vi "XY Graph Plot Convolution Dialog.vi"(6 "Reference Decay":cluster{"t Array":dbl[], "I Array":dbl[]}, 8 "Error In":errorcluster, 9 "Valid Reference Decay?":bool, 10 "Plot at Coordinates":i32, 11 "XY Graph":refnum<vi>) -> (0 "Error Out":errorcluster, 1 "Plot Destination out":T4, 2 "Convolution Product Options out":T1 {"Plot 2" items=["M0_H00_000: Plot", "M0_H00_020: Plot"]; "Plot 1" items=["M0_H00_000: Plot", "M0_H00_020: Plot"]}, 3 "XY Graph (dup)":refnum<vi>, 4 "Cancelled":bool)   [LabVIEW 2021, in "XY Graph Add-Ons.lvlib"]
uses:
  Plot Destination.ctl
  XY Graph Convolution Product Options.ctl
  XY Graph Convolution Period Type.ctl
  XY Graph Convolution Step Type.ctl
  XY Graph Add-Ons.lvlib
  Graphs.lvlib
panel:
  in  "Convolution Product Options":T1 {"Step" min=0.0; "Period" min=0.0; "Plot 2" items=["Extrapolated M0 IRF", "M0_H00_000: Liver", "2-Exp Fit of M0_H00_000: Liver", "2-Exp Fit of M0_H00_000: Liver Residuals", "M0_H00_001: Liver", "2-Exp Fit of M0_H00_001: Liver", "2-Exp Fit of M0_H00_001: Liver Residuals", "M0_H00_002: Liver", "2-Exp Fit of M0_H00_002: Liver", "2-Exp Fit of M0_H00_002: Liver Residuals", "M0_H00_003: Liver", "2-Exp Fit of M0_H00_003: Liver", "2-Exp Fit of M0_H00_003: Liver Residuals", "M0_H00_004: Liver", "2-Exp Fit of M0_H00_004: Liver", "2-Exp Fit of M0_H00_004: Liver Residuals", "M0_H00_005: Liver", "2-Exp Fit of M0_H00_005: Liver", "2-Exp Fit of M0_H00_005: Liver Residuals", "M0_H00_006: Liver", "2-Exp Fit of M0_H00_006: Liver", "2-Exp Fit of M0_H00_006: Liver Residuals", "M0_H00_007: Liver", "2-Exp Fit of M0_H00_007: Liver", "2-Exp Fit of M0_H00_007: Liver Residuals", "M0_H00_008: Liver", "2-Exp Fit of M0_H00_008: Liver", "2-Exp Fit of M0_H00_008: Liver Residuals", "M0_H00_009: Liver", "2-Exp Fit of M0_H00_009: Liver", "2-Exp Fit of M0_H00_009: Liver Residuals", "M0_H00_010: Liver", "2-Exp Fit of M0_H00_010: Liver", "2-Exp Fit of M0_H00_010: Liver Residuals", "M0_H00_011: Liver", "2-Exp Fit of M0_H00_011: Liver", "2-Exp Fit of M0_H00_011: Liver Residuals", "M0_H00_012: Liver", "2-Exp Fit of M0_H00_012: Liver", "2-Exp Fit of M0_H00_012: Liver Residuals", "M0_H00_013: Liver", "2-Exp Fit of M0_H00_013: Liver", "2-Exp Fit of M0_H00_013: Liver Residuals", "M0_H00_014: Liver", "2-Exp Fit of M0_H00_014: Liver", "2-Exp Fit of M0_H00_014: Liver Residuals", "M0_H00_015: Liver", "2-Exp Fit of M0_H00_015: Liver", "2-Exp Fit of M0_H00_015: Liver Residuals", "M0_H00_016: Liver", "2-Exp Fit of M0_H00_016: Liver", "2-Exp Fit of M0_H00_016: Liver Residuals", "M0_H00_017: Liver", "2-Exp Fit of M0_H00_017: Liver", "2-Exp Fit of M0_H00_017: Liver Residuals", "M0_H00_018: Liver", "2-Exp Fit of M0_H00_018: Liver", "2-Exp Fit of M0_H00_018: Liver Residuals", "M0_H00_019: Liver", "2-Exp Fit of M0_H00_019: Liver", "2-Exp Fit of M0_H00_019: Liver Residuals", "M0_H00_020: Liver", "2-Exp Fit of M0_H00_020: Liver", "2-Exp Fit of M0_H00_020: Liver Residuals", "M0_H00_021: Liver", "2-Exp Fit of M0_H00_021: Liver", "2-Exp Fit of M0_H00_021: Liver Residuals", "M0_H00_022: Liver", "2-Exp Fit of M0_H00_022: Liver", "2-Exp Fit of M0_H00_022: Liver Residuals", "M0_H00_023: Liver", "2-Exp Fit of M0_H00_023: Liver", "2-Exp Fit of M0_H00_023: Liver Residuals", "M0_H00_024: Liver", "2-Exp Fit of M0_H00_024: Liver", "2-Exp Fit of M0_H00_024: Liver Residuals", "M0_H00_025: Liver", "2-Exp Fit of M0_H00_025: Liver", "2-Exp Fit of M0_H00_025: Liver Residuals", "M0_H00_026: Liver", "2-Exp Fit of M0_H00_026: Liver", "2-Exp Fit of M0_H00_026: Liver Residuals", "M0_H00_027: Liver", "2-Exp Fit of M0_H00_027: Liver", "2-Exp Fit of M0_H00_027: Liver Residuals", "M0_H00_028: Liver", "2-Exp Fit of M0_H00_028: Liver", "2-Exp Fit of M0_H00_028: Liver Residuals", "M0_H00_029: Liver", "2-Exp Fit of M0_H00_029: Liver", "2-Exp Fit of M0_H00_029: Liver Residuals", "M0_H00_030: Liver", "2-Exp Fit of M0_H00_030: Liver", "2-Exp Fit of M0_H00_030: Liver Residuals", "M0_H00_031: Liver", "2-Exp Fit of M0_H00_031: Liver", "2-Exp Fit of M0_H00_031: Liver Residuals", "M0_H00_032: Liver", "2-Exp Fit of M0_H00_032: Liver", "2-Exp Fit of M0_H00_032: Liver Residuals", "M0_H00_033: Liver", "2-Exp Fit of M0_H00_033: Liver", "2-Exp Fit of M0_H00_033: Liver Residuals", "M0_H00_034: Liver", "2-Exp Fit of M0_H00_034: Liver", "2-Exp Fit of M0_H00_034: Liver Residuals", "M0_H00_035: Liver", "2-Exp Fit of M0_H00_035: Liver", "2-Exp Fit of M0_H00_035: Liver Residuals", "M0_H00_036: Liver", "2-Exp Fit of M0_H00_036: Liver", "2-Exp Fit of M0_H00_036: Liver Residuals", "M0_H00_037: Liver", "2-Exp Fit of M0_H00_037: Liver", "2-Exp Fit of M0_H00_037: Liver Residuals", "M0_H00_038: Liver", "2-Exp Fit of M0_H00_038: Liver", "2-Exp Fit of M0_H00_038: Liver Residuals", "M0_H00_039: Liver", "2-Exp Fit of M0_H00_039: Liver", "2-Exp Fit of M0_H00_039: Liver Residuals", "M0_H00_040: Liver", "2-Exp Fit of M0_H00_040: Liver", "2-Exp Fit of M0_H00_040: Liver Residuals", "M0_H00_041: Liver", "2-Exp Fit of M0_H00_041: Liver", "2-Exp Fit of M0_H00_041: Liver Residuals", "M0_H00_042: Liver", "2-Exp Fit of M0_H00_042: Liver", "2-Exp Fit of M0_H00_042: Liver Residuals", "M0_H00_043: Liver", "2-Exp Fit of M0_H00_043: Liver", "2-Exp Fit of M0_H00_043: Liver Residuals", "M0_H00_044: Liver", "2-Exp Fit of M0_H00_044: Liver", "2-Exp Fit of M0_H00_044: Liver Residuals", "M0_H00_045: Liver", "2-Exp Fit of M0_H00_045: Liver", "2-Exp Fit of M0_H00_045: Liver Residuals", "M0_H00_046: Liver", "2-Exp Fit of M0_H00_046: Liver", "2-Exp Fit of M0_H00_046: Liver Residuals", "M0_H00_047: Liver", "2-Exp Fit of M0_H00_047: Liver", "2-Exp Fit of M0_H00_047: Liver Residuals", "M0_H00_048: Liver", "2-Exp Fit of M0_H00_048: Liver", "2-Exp Fit of M0_H00_048: Liver Residuals", "M0_H00_049: Liver", "2-Exp Fit of M0_H00_049: Liver", "2-Exp Fit of M0_H00_049: Liver Residuals", "M0_H00_050: Liver", "2-Exp Fit of M0_H00_050: Liver", "2-Exp Fit of M0_H00_050: Liver Residuals", "M0_H00_051: Liver", "2-Exp Fit of M0_H00_051: Liver", "2-Exp Fit of M0_H00_051: Liver Residuals", "M0_H00_052: Liver", "2-Exp Fit of M0_H00_052: Liver", "2-Exp Fit of M0_H00_052: Liver Residuals", "M0_H00_053: Liver", "2-Exp Fit of M0_H00_053: Liver", "2-Exp Fit of M0_H00_053: Liver Residuals", "M0_H00_054: Liver", "2-Exp Fit of M0_H00_054: Liver", "2-Exp Fit of M0_H00_054: Liver Residuals", "M0_H00_055: Liver", "2-Exp Fit of M0_H00_055: Liver", "2-Exp Fit of M0_H00_055: Liver Residuals", "M0_H00_056: Liver", "2-Exp Fit of M0_H00_056: Liver", "2-Exp Fit of M0_H00_056: Liver Residuals", "M0_H00_057: Liver", "2-Exp Fit of M0_H00_057: Liver", "2-Exp Fit of M0_H00_057: Liver Residuals", "M0_H00_058: Liver", "2-Exp Fit of M0_H00_058: Liver", "2-Exp Fit of M0_H00_058: Liver Residuals", "M0_H00_059: Liver", "2-Exp Fit of M0_H00_059: Liver", "2-Exp Fit of M0_H00_059: Liver Residuals", "M0_H00_060: Liver", "2-Exp Fit of M0_H00_060: Liver", "2-Exp Fit of M0_H00_060: Liver Residuals", "M0_H00_061: Liver", "2-Exp Fit of M0_H00_061: Liver", "2-Exp Fit of M0_H00_061: Liver Residuals", "M0_H00_062: Liver", "2-Exp Fit of M0_H00_062: Liver", "2-Exp Fit of M0_H00_062: Liver Residuals", "M0_H00_063: Liver", "2-Exp Fit of M0_H00_063: Liver", "2-Exp Fit of M0_H00_063: Liver Residuals", "M0_H00_064: Liver", "2-Exp Fit of M0_H00_064: Liver", "2-Exp Fit of M0_H00_064: Liver Residuals", "M0_H00_065: Liver", "2-Exp Fit of M0_H00_065: Liver", "2-Exp Fit of M0_H00_065: Liver Residuals", "M0_H00_066: Liver", "2-Exp Fit of M0_H00_066: Liver", "2-Exp Fit of M0_H00_066: Liver Residuals", "M0_H00_067: Liver", "2-Exp Fit of M0_H00_067: Liver", "2-Exp Fit of M0_H00_067: Liver Residuals", "M0_H00_068: Liver", "2-Exp Fit of M0_H00_068: Liver", "2-Exp Fit of M0_H00_068: Liver Residuals", "M0_H00_069: Liver", "2-Exp Fit of M0_H00_069: Liver", "2-Exp Fit of M0_H00_069: Liver Residuals", "M0_H00_070: Liver", "2-Exp Fit of M0_H00_070: Liver", "2-Exp Fit of M0_H00_070: Liver Residuals", "M0_H00_071: Liver", "2-Exp Fit of M0_H00_071: Liver", "2-Exp Fit of M0_H00_071: Liver Residuals", "M0_H00_072: Liver", "2-Exp Fit of M0_H00_072: Liver", "2-Exp Fit of M0_H00_072: Liver Residuals", "M0_H00_073: Liver", "2-Exp Fit of M0_H00_073: Liver", "2-Exp Fit of M0_H00_073: Liver Residuals", "M0_H00_074: Liver", "2-Exp Fit of M0_H00_074: Liver", "2-Exp Fit of M0_H00_074: Liver Residuals", "M0_H00_075: Liver", "2-Exp Fit of M0_H00_075: Liver", "2-Exp Fit of M0_H00_075: Liver Residuals", "M0_H00_076: Liver", "2-Exp Fit of M0_H00_076: Liver", "2-Exp Fit of M0_H00_076: Liver Residuals", "M0_H00_077: Liver", "2-Exp Fit of M0_H00_077: Liver", "2-Exp Fit of M0_H00_077: Liver Residuals", "M0_H00_078: Liver", "2-Exp Fit of M0_H00_078: Liver", "2-Exp Fit of M0_H00_078: Liver Residuals", "M0_H00_079: Liver", "2-Exp Fit of M0_H00_079: Liver", "2-Exp Fit of M0_H00_079: Liver Residuals", "M0_H00_080: Liver", "2-Exp Fit of M0_H00_080: Liver", "2-Exp Fit of M0_H00_080: Liver Residuals", "M0_H00_081: Liver", "2-Exp Fit of M0_H00_081: Liver", "2-Exp Fit of M0_H00_081: Liver Residuals", "M0_H00_082: Liver", "2-Exp Fit of M0_H00_082: Liver", "2-Exp Fit of M0_H00_082: Liver Residuals", "M0_H00_083: Liver", "2-Exp Fit of M0_H00_083: Liver", "2-Exp Fit of M0_H00_083: Liver Residuals", "M0_H00_084: Liver", "2-Exp Fit of M0_H00_084: Liver", "2-Exp Fit of M0_H00_084: Liver Residuals", "M0_H00_085: Liver", "2-Exp Fit of M0_H00_085: Liver", "2-Exp Fit of M0_H00_085: Liver Residuals", "M0_H00_086: Liver", "2-Exp Fit of M0_H00_086: Liver", "2-Exp Fit of M0_H00_086: Liver Residuals", "M0_H00_087: Liver", "2-Exp Fit of M0_H00_087: Liver", "2-Exp Fit of M0_H00_087: Liver Residuals", "M0_H00_088: Liver", "2-Exp Fit of M0_H00_088: Liver", "2-Exp Fit of M0_H00_088: Liver Residuals", "M0_H00_089: Liver", "2-Exp Fit of M0_H00_089: Liver", "2-Exp Fit of M0_H00_089: Liver Residuals", "M0_H00_090: Liver", "2-Exp Fit of M0_H00_090: Liver", "2-Exp Fit of M0_H00_090: Liver Residuals", "M0_H00_091: Liver", "2-Exp Fit of M0_H00_091: Liver", "2-Exp Fit of M0_H00_091: Liver Residuals", "M0_H00_092: Liver", "2-Exp Fit of M0_H00_092: Liver", "2-Exp Fit of M0_H00_092: Liver Residuals", "M0_H00_093: Liver", "2-Exp Fit of M0_H00_093: Liver", "2-Exp Fit of M0_H00_093: Liver Residuals", "M0_H00_094: Liver", "2-Exp Fit of M0_H00_094: Liver", "2-Exp Fit of M0_H00_094: Liver Residuals", "M0_H00_095: Liver", "2-Exp Fit of M0_H00_095: Liver", "2-Exp Fit of M0_H00_095: Liver Residuals", "M0_H00_096: Liver", "2-Exp Fit of M0_H00_096: Liver", "2-Exp Fit of M0_H00_096: Liver Residuals", "M0_H00_097: Liver", "2-Exp Fit of M0_H00_097: Liver", "2-Exp Fit of M0_H00_097: Liver Residuals", "M0_H00_098: Liver", "2-Exp Fit of M0_H00_098: Liver", "2-Exp Fit of M0_H00_098: Liver Residuals", "M0_H00_099: Liver", "2-Exp Fit of M0_H00_099: Liver", "2-Exp Fit of M0_H00_099: Liver Residuals", "M0_H00_100: Liver", "2-Exp Fit of M0_H00_100: Liver", "2-Exp Fit of M0_H00_100: Liver Residuals", "M0_H00_101: Liver", "2-Exp Fit of M0_H00_101: Liver", "2-Exp Fit of M0_H00_101: Liver Residuals", "M0_H00_102: Liver", "2-Exp Fit of M0_H00_102: Liver", "2-Exp Fit of M0_H00_102: Liver Residuals", "M0_H00_103: Liver", "2-Exp Fit of M0_H00_103: Liver", "2-Exp Fit of M0_H00_103: Liver Residuals", "M0_H00_104: Liver", "2-Exp Fit of M0_H00_104: Liver", "2-Exp Fit of M0_H00_104: Liver Residuals", "M0_H00_105: Liver", "2-Exp Fit of M0_H00_105: Liver", "2-Exp Fit of M0_H00_105: Liver Residuals", "M0_H00_106: Liver", "2-Exp Fit of M0_H00_106: Liver", "2-Exp Fit of M0_H00_106: Liver Residuals", "M0_H00_107: Liver", "2-Exp Fit of M0_H00_107: Liver", "2-Exp Fit of M0_H00_107: Liver Residuals", "M0_H00_108: Liver", "2-Exp Fit of M0_H00_108: Liver", "2-Exp Fit of M0_H00_108: Liver Residuals", "M0_H00_109: Liver", "2-Exp Fit of M0_H00_109: Liver", "2-Exp Fit of M0_H00_109: Liver Residuals", "M0_H00_110: Liver", "2-Exp Fit of M0_H00_110: Liver", "2-Exp Fit of M0_H00_110: Liver Residuals", "M0_H00_111: Liver", "2-Exp Fit of M0_H00_111: Liver", "2-Exp Fit of M0_H00_111: Liver Residuals", "M0_H00_112: Liver", "2-Exp Fit of M0_H00_112: Liver", "2-Exp Fit of M0_H00_112: Liver Residuals", "M0_H00_113: Liver", "2-Exp Fit of M0_H00_113: Liver", "2-Exp Fit of M0_H00_113: Liver Residuals", "M0_H00_114: Liver", "2-Exp Fit of M0_H00_114: Liver", "2-Exp Fit of M0_H00_114: Liver Residuals", "M0_H00_115: Liver", "2-Exp Fit of M0_H00_115: Liver", "2-Exp Fit of M0_H00_115: Liver Residuals", "M0_H00_116: Liver", "2-Exp Fit of M0_H00_116: Liver", "2-Exp Fit of M0_H00_116: Liver Residuals", "M0_H00_117: Liver", "2-Exp Fit of M0_H00_117: Liver", "2-Exp Fit of M0_H00_117: Liver Residuals", "M0_H00_118: Liver", "2-Exp Fit of M0_H00_118: Liver", "2-Exp Fit of M0_H00_118: Liver Residuals", "M0_H00_119: Liver", "2-Exp Fit of M0_H00_119: Liver", "2-Exp Fit of M0_H00_119: Liver Residuals", "M0_H00_120: Liver", "2-Exp Fit of M0_H00_120: Liver", "2-Exp Fit of M0_H00_120: Liver Residuals", "M0_H00_121: Liver", "2-Exp Fit of M0_H00_121: Liver", "2-Exp Fit of M0_H00_121: Liver Residuals", "M0_H00_122: Liver", "2-Exp Fit of M0_H00_122: Liver", "2-Exp Fit of M0_H00_122: Liver Residuals", "M0_H00_123: Liver", "2-Exp Fit of M0_H00_123: Liver", "2-Exp Fit of M0_H00_123: Liver Residuals", "M0_H00_124: Liver", "2-Exp Fit of M0_H00_124: Liver", "2-Exp Fit of M0_H00_124: Liver Residuals", "M0_H00_125: Liver", "2-Exp Fit of M0_H00_125: Liver", "2-Exp Fit of M0_H00_125: Liver Residuals", "M0_H00_126: Liver", "2-Exp Fit of M0_H00_126: Liver", "2-Exp Fit of M0_H00_126: Liver Residuals", "M0_H00_127: Liver", "2-Exp Fit of M0_H00_127: Liver", "2-Exp Fit of M0_H00_127: Liver Residuals", "M0_H00_128: Liver", "2-Exp Fit of M0_H00_128: Liver", "2-Exp Fit of M0_H00_128: Liver Residuals", "M0_H00_129: Liver", "2-Exp Fit of M0_H00_129: Liver", "2-Exp Fit of M0_H00_129: Liver Residuals", "M0_H00_130: Liver", "2-Exp Fit of M0_H00_130: Liver", "2-Exp Fit of M0_H00_130: Liver Residuals", "M0_H00_131: Liver", "2-Exp Fit of M0_H00_131: Liver", "2-Exp Fit of M0_H00_131: Liver Residuals", "M0_H00_132: Liver", "2-Exp Fit of M0_H00_132: Liver", "2-Exp Fit of M0_H00_132: Liver Residuals", "M0_H00_133: Liver", "2-Exp Fit of M0_H00_133: Liver", "2-Exp Fit of M0_H00_133: Liver Residuals", "M0_H00_134: Liver", "2-Exp Fit of M0_H00_134: Liver", "2-Exp Fit of M0_H00_134: Liver Residuals", "M0_H00_135: Liver", "2-Exp Fit of M0_H00_135: Liver", "2-Exp Fit of M0_H00_135: Liver Residuals", "M0_H00_136: Liver", "2-Exp Fit of M0_H00_136: Liver", "2-Exp Fit of M0_H00_136: Liver Residuals", "M0_H00_137: Liver", "2-Exp Fit of M0_H00_137: Liver", "2-Exp Fit of M0_H00_137: Liver Residuals", "M0_H00_138: Liver", "2-Exp Fit of M0_H00_138: Liver", "2-Exp Fit of M0_H00_138: Liver Residuals", "M0_H00_139: Liver", "2-Exp Fit of M0_H00_139: Liver", "2-Exp Fit of M0_H00_139: Liver Residuals", "M0_H00_140: Liver", "2-Exp Fit of M0_H00_140: Liver", "2-Exp Fit of M0_H00_140: Liver Residuals", "M0_H00_141: Liver", "2-Exp Fit of M0_H00_141: Liver", "2-Exp Fit of M0_H00_141: Liver Residuals", "M0_H00_142: Liver", "2-Exp Fit of M0_H00_142: Liver", "2-Exp Fit of M0_H00_142: Liver Residuals", "M0_H00_143: Liver", "2-Exp Fit of M0_H00_143: Liver", "2-Exp Fit of M0_H00_143: Liver Residuals", "M0_H00_144: Liver", "2-Exp Fit of M0_H00_144: Liver", "2-Exp Fit of M0_H00_144: Liver Residuals", "M0_H00_145: Liver", "2-Exp Fit of M0_H00_145: Liver", "2-Exp Fit of M0_H00_145: Liver Residuals", "M0_H00_146: Liver", "2-Exp Fit of M0_H00_146: Liver", "2-Exp Fit of M0_H00_146: Liver Residuals", "M0_H00_147: Liver", "2-Exp Fit of M0_H00_147: Liver", "2-Exp Fit of M0_H00_147: Liver Residuals", "M0_H00_148: Liver", "2-Exp Fit of M0_H00_148: Liver", "2-Exp Fit of M0_H00_148: Liver Residuals", "M0_H00_149: Liver", "2-Exp Fit of M0_H00_149: Liver", "2-Exp Fit of M0_H00_149: Liver Residuals", "M0_H00_150: Liver", "2-Exp Fit of M0_H00_150: Liver", "2-Exp Fit of M0_H00_150: Liver Residuals", "M0_H00_151: Liver", "2-Exp Fit of M0_H00_151: Liver", "2-Exp Fit of M0_H00_151: Liver Residuals", "M0_H00_152: Liver", "2-Exp Fit of M0_H00_152: Liver", "2-Exp Fit of M0_H00_152: Liver Residuals", "M0_H00_153: Liver", "2-Exp Fit of M0_H00_153: Liver", "2-Exp Fit of M0_H00_153: Liver Residuals", "M0_H00_154: Liver", "2-Exp Fit of M0_H00_154: Liver", "2-Exp Fit of M0_H00_154: Liver Residuals", "M0_H00_155: Liver", "2-Exp Fit of M0_H00_155: Liver", "2-Exp Fit of M0_H00_155: Liver Residuals", "M0_H00_156: Liver", "2-Exp Fit of M0_H00_156: Liver", "2-Exp Fit of M0_H00_156: Liver Residuals", "M0_H00_157: Liver", "2-Exp Fit of M0_H00_157: Liver", "2-Exp Fit of M0_H00_157: Liver Residuals", "M0_H00_158: Liver", "2-Exp Fit of M0_H00_158: Liver", "2-Exp Fit of M0_H00_158: Liver Residuals", "M0_H00_159: Liver", "2-Exp Fit of M0_H00_159: Liver", "2-Exp Fit of M0_H00_159: Liver Residuals", "M0_H00_160: Liver", "2-Exp Fit of M0_H00_160: Liver", "2-Exp Fit of M0_H00_160: Liver Residuals", "M0_H00_161: Liver", "2-Exp Fit of M0_H00_161: Liver", "2-Exp Fit of M0_H00_161: Liver Residuals", "M0_H00_162: Liver", "2-Exp Fit of M0_H00_162: Liver", "2-Exp Fit of M0_H00_162: Liver Residuals", "M0_H00_163: Liver", "2-Exp Fit of M0_H00_163: Liver", "2-Exp Fit of M0_H00_163: Liver Residuals", "M0_H00_164: Liver", "2-Exp Fit of M0_H00_164: Liver", "2-Exp Fit of M0_H00_164: Liver Residuals", "-", "IRF/Reference Decay"]; "Plot 1" items=["Extrapolated M0 IRF", "M0_H00_000: Liver", "2-Exp Fit of M0_H00_000: Liver", "2-Exp Fit of M0_H00_000: Liver Residuals", "M0_H00_001: Liver", "2-Exp Fit of M0_H00_001: Liver", "2-Exp Fit of M0_H00_001: Liver Residuals", "M0_H00_002: Liver", "2-Exp Fit of M0_H00_002: Liver", "2-Exp Fit of M0_H00_002: Liver Residuals", "M0_H00_003: Liver", "2-Exp Fit of M0_H00_003: Liver", "2-Exp Fit of M0_H00_003: Liver Residuals", "M0_H00_004: Liver", "2-Exp Fit of M0_H00_004: Liver", "2-Exp Fit of M0_H00_004: Liver Residuals", "M0_H00_005: Liver", "2-Exp Fit of M0_H00_005: Liver", "2-Exp Fit of M0_H00_005: Liver Residuals", "M0_H00_006: Liver", "2-Exp Fit of M0_H00_006: Liver", "2-Exp Fit of M0_H00_006: Liver Residuals", "M0_H00_007: Liver", "2-Exp Fit of M0_H00_007: Liver", "2-Exp Fit of M0_H00_007: Liver Residuals", "M0_H00_008: Liver", "2-Exp Fit of M0_H00_008: Liver", "2-Exp Fit of M0_H00_008: Liver Residuals", "M0_H00_009: Liver", "2-Exp Fit of M0_H00_009: Liver", "2-Exp Fit of M0_H00_009: Liver Residuals", "M0_H00_010: Liver", "2-Exp Fit of M0_H00_010: Liver", "2-Exp Fit of M0_H00_010: Liver Residuals", "M0_H00_011: Liver", "2-Exp Fit of M0_H00_011: Liver", "2-Exp Fit of M0_H00_011: Liver Residuals", "M0_H00_012: Liver", "2-Exp Fit of M0_H00_012: Liver", "2-Exp Fit of M0_H00_012: Liver Residuals", "M0_H00_013: Liver", "2-Exp Fit of M0_H00_013: Liver", "2-Exp Fit of M0_H00_013: Liver Residuals", "M0_H00_014: Liver", "2-Exp Fit of M0_H00_014: Liver", "2-Exp Fit of M0_H00_014: Liver Residuals", "M0_H00_015: Liver", "2-Exp Fit of M0_H00_015: Liver", "2-Exp Fit of M0_H00_015: Liver Residuals", "M0_H00_016: Liver", "2-Exp Fit of M0_H00_016: Liver", "2-Exp Fit of M0_H00_016: Liver Residuals", "M0_H00_017: Liver", "2-Exp Fit of M0_H00_017: Liver", "2-Exp Fit of M0_H00_017: Liver Residuals", "M0_H00_018: Liver", "2-Exp Fit of M0_H00_018: Liver", "2-Exp Fit of M0_H00_018: Liver Residuals", "M0_H00_019: Liver", "2-Exp Fit of M0_H00_019: Liver", "2-Exp Fit of M0_H00_019: Liver Residuals", "M0_H00_020: Liver", "2-Exp Fit of M0_H00_020: Liver", "2-Exp Fit of M0_H00_020: Liver Residuals", "M0_H00_021: Liver", "2-Exp Fit of M0_H00_021: Liver", "2-Exp Fit of M0_H00_021: Liver Residuals", "M0_H00_022: Liver", "2-Exp Fit of M0_H00_022: Liver", "2-Exp Fit of M0_H00_022: Liver Residuals", "M0_H00_023: Liver", "2-Exp Fit of M0_H00_023: Liver", "2-Exp Fit of M0_H00_023: Liver Residuals", "M0_H00_024: Liver", "2-Exp Fit of M0_H00_024: Liver", "2-Exp Fit of M0_H00_024: Liver Residuals", "M0_H00_025: Liver", "2-Exp Fit of M0_H00_025: Liver", "2-Exp Fit of M0_H00_025: Liver Residuals", "M0_H00_026: Liver", "2-Exp Fit of M0_H00_026: Liver", "2-Exp Fit of M0_H00_026: Liver Residuals", "M0_H00_027: Liver", "2-Exp Fit of M0_H00_027: Liver", "2-Exp Fit of M0_H00_027: Liver Residuals", "M0_H00_028: Liver", "2-Exp Fit of M0_H00_028: Liver", "2-Exp Fit of M0_H00_028: Liver Residuals", "M0_H00_029: Liver", "2-Exp Fit of M0_H00_029: Liver", "2-Exp Fit of M0_H00_029: Liver Residuals", "M0_H00_030: Liver", "2-Exp Fit of M0_H00_030: Liver", "2-Exp Fit of M0_H00_030: Liver Residuals", "M0_H00_031: Liver", "2-Exp Fit of M0_H00_031: Liver", "2-Exp Fit of M0_H00_031: Liver Residuals", "M0_H00_032: Liver", "2-Exp Fit of M0_H00_032: Liver", "2-Exp Fit of M0_H00_032: Liver Residuals", "M0_H00_033: Liver", "2-Exp Fit of M0_H00_033: Liver", "2-Exp Fit of M0_H00_033: Liver Residuals", "M0_H00_034: Liver", "2-Exp Fit of M0_H00_034: Liver", "2-Exp Fit of M0_H00_034: Liver Residuals", "M0_H00_035: Liver", "2-Exp Fit of M0_H00_035: Liver", "2-Exp Fit of M0_H00_035: Liver Residuals", "M0_H00_036: Liver", "2-Exp Fit of M0_H00_036: Liver", "2-Exp Fit of M0_H00_036: Liver Residuals", "M0_H00_037: Liver", "2-Exp Fit of M0_H00_037: Liver", "2-Exp Fit of M0_H00_037: Liver Residuals", "M0_H00_038: Liver", "2-Exp Fit of M0_H00_038: Liver", "2-Exp Fit of M0_H00_038: Liver Residuals", "M0_H00_039: Liver", "2-Exp Fit of M0_H00_039: Liver", "2-Exp Fit of M0_H00_039: Liver Residuals", "M0_H00_040: Liver", "2-Exp Fit of M0_H00_040: Liver", "2-Exp Fit of M0_H00_040: Liver Residuals", "M0_H00_041: Liver", "2-Exp Fit of M0_H00_041: Liver", "2-Exp Fit of M0_H00_041: Liver Residuals", "M0_H00_042: Liver", "2-Exp Fit of M0_H00_042: Liver", "2-Exp Fit of M0_H00_042: Liver Residuals", "M0_H00_043: Liver", "2-Exp Fit of M0_H00_043: Liver", "2-Exp Fit of M0_H00_043: Liver Residuals", "M0_H00_044: Liver", "2-Exp Fit of M0_H00_044: Liver", "2-Exp Fit of M0_H00_044: Liver Residuals", "M0_H00_045: Liver", "2-Exp Fit of M0_H00_045: Liver", "2-Exp Fit of M0_H00_045: Liver Residuals", "M0_H00_046: Liver", "2-Exp Fit of M0_H00_046: Liver", "2-Exp Fit of M0_H00_046: Liver Residuals", "M0_H00_047: Liver", "2-Exp Fit of M0_H00_047: Liver", "2-Exp Fit of M0_H00_047: Liver Residuals", "M0_H00_048: Liver", "2-Exp Fit of M0_H00_048: Liver", "2-Exp Fit of M0_H00_048: Liver Residuals", "M0_H00_049: Liver", "2-Exp Fit of M0_H00_049: Liver", "2-Exp Fit of M0_H00_049: Liver Residuals", "M0_H00_050: Liver", "2-Exp Fit of M0_H00_050: Liver", "2-Exp Fit of M0_H00_050: Liver Residuals", "M0_H00_051: Liver", "2-Exp Fit of M0_H00_051: Liver", "2-Exp Fit of M0_H00_051: Liver Residuals", "M0_H00_052: Liver", "2-Exp Fit of M0_H00_052: Liver", "2-Exp Fit of M0_H00_052: Liver Residuals", "M0_H00_053: Liver", "2-Exp Fit of M0_H00_053: Liver", "2-Exp Fit of M0_H00_053: Liver Residuals", "M0_H00_054: Liver", "2-Exp Fit of M0_H00_054: Liver", "2-Exp Fit of M0_H00_054: Liver Residuals", "M0_H00_055: Liver", "2-Exp Fit of M0_H00_055: Liver", "2-Exp Fit of M0_H00_055: Liver Residuals", "M0_H00_056: Liver", "2-Exp Fit of M0_H00_056: Liver", "2-Exp Fit of M0_H00_056: Liver Residuals", "M0_H00_057: Liver", "2-Exp Fit of M0_H00_057: Liver", "2-Exp Fit of M0_H00_057: Liver Residuals", "M0_H00_058: Liver", "2-Exp Fit of M0_H00_058: Liver", "2-Exp Fit of M0_H00_058: Liver Residuals", "M0_H00_059: Liver", "2-Exp Fit of M0_H00_059: Liver", "2-Exp Fit of M0_H00_059: Liver Residuals", "M0_H00_060: Liver", "2-Exp Fit of M0_H00_060: Liver", "2-Exp Fit of M0_H00_060: Liver Residuals", "M0_H00_061: Liver", "2-Exp Fit of M0_H00_061: Liver", "2-Exp Fit of M0_H00_061: Liver Residuals", "M0_H00_062: Liver", "2-Exp Fit of M0_H00_062: Liver", "2-Exp Fit of M0_H00_062: Liver Residuals", "M0_H00_063: Liver", "2-Exp Fit of M0_H00_063: Liver", "2-Exp Fit of M0_H00_063: Liver Residuals", "M0_H00_064: Liver", "2-Exp Fit of M0_H00_064: Liver", "2-Exp Fit of M0_H00_064: Liver Residuals", "M0_H00_065: Liver", "2-Exp Fit of M0_H00_065: Liver", "2-Exp Fit of M0_H00_065: Liver Residuals", "M0_H00_066: Liver", "2-Exp Fit of M0_H00_066: Liver", "2-Exp Fit of M0_H00_066: Liver Residuals", "M0_H00_067: Liver", "2-Exp Fit of M0_H00_067: Liver", "2-Exp Fit of M0_H00_067: Liver Residuals", "M0_H00_068: Liver", "2-Exp Fit of M0_H00_068: Liver", "2-Exp Fit of M0_H00_068: Liver Residuals", "M0_H00_069: Liver", "2-Exp Fit of M0_H00_069: Liver", "2-Exp Fit of M0_H00_069: Liver Residuals", "M0_H00_070: Liver", "2-Exp Fit of M0_H00_070: Liver", "2-Exp Fit of M0_H00_070: Liver Residuals", "M0_H00_071: Liver", "2-Exp Fit of M0_H00_071: Liver", "2-Exp Fit of M0_H00_071: Liver Residuals", "M0_H00_072: Liver", "2-Exp Fit of M0_H00_072: Liver", "2-Exp Fit of M0_H00_072: Liver Residuals", "M0_H00_073: Liver", "2-Exp Fit of M0_H00_073: Liver", "2-Exp Fit of M0_H00_073: Liver Residuals", "M0_H00_074: Liver", "2-Exp Fit of M0_H00_074: Liver", "2-Exp Fit of M0_H00_074: Liver Residuals", "M0_H00_075: Liver", "2-Exp Fit of M0_H00_075: Liver", "2-Exp Fit of M0_H00_075: Liver Residuals", "M0_H00_076: Liver", "2-Exp Fit of M0_H00_076: Liver", "2-Exp Fit of M0_H00_076: Liver Residuals", "M0_H00_077: Liver", "2-Exp Fit of M0_H00_077: Liver", "2-Exp Fit of M0_H00_077: Liver Residuals", "M0_H00_078: Liver", "2-Exp Fit of M0_H00_078: Liver", "2-Exp Fit of M0_H00_078: Liver Residuals", "M0_H00_079: Liver", "2-Exp Fit of M0_H00_079: Liver", "2-Exp Fit of M0_H00_079: Liver Residuals", "M0_H00_080: Liver", "2-Exp Fit of M0_H00_080: Liver", "2-Exp Fit of M0_H00_080: Liver Residuals", "M0_H00_081: Liver", "2-Exp Fit of M0_H00_081: Liver", "2-Exp Fit of M0_H00_081: Liver Residuals", "M0_H00_082: Liver", "2-Exp Fit of M0_H00_082: Liver", "2-Exp Fit of M0_H00_082: Liver Residuals", "M0_H00_083: Liver", "2-Exp Fit of M0_H00_083: Liver", "2-Exp Fit of M0_H00_083: Liver Residuals", "M0_H00_084: Liver", "2-Exp Fit of M0_H00_084: Liver", "2-Exp Fit of M0_H00_084: Liver Residuals", "M0_H00_085: Liver", "2-Exp Fit of M0_H00_085: Liver", "2-Exp Fit of M0_H00_085: Liver Residuals", "M0_H00_086: Liver", "2-Exp Fit of M0_H00_086: Liver", "2-Exp Fit of M0_H00_086: Liver Residuals", "M0_H00_087: Liver", "2-Exp Fit of M0_H00_087: Liver", "2-Exp Fit of M0_H00_087: Liver Residuals", "M0_H00_088: Liver", "2-Exp Fit of M0_H00_088: Liver", "2-Exp Fit of M0_H00_088: Liver Residuals", "M0_H00_089: Liver", "2-Exp Fit of M0_H00_089: Liver", "2-Exp Fit of M0_H00_089: Liver Residuals", "M0_H00_090: Liver", "2-Exp Fit of M0_H00_090: Liver", "2-Exp Fit of M0_H00_090: Liver Residuals", "M0_H00_091: Liver", "2-Exp Fit of M0_H00_091: Liver", "2-Exp Fit of M0_H00_091: Liver Residuals", "M0_H00_092: Liver", "2-Exp Fit of M0_H00_092: Liver", "2-Exp Fit of M0_H00_092: Liver Residuals", "M0_H00_093: Liver", "2-Exp Fit of M0_H00_093: Liver", "2-Exp Fit of M0_H00_093: Liver Residuals", "M0_H00_094: Liver", "2-Exp Fit of M0_H00_094: Liver", "2-Exp Fit of M0_H00_094: Liver Residuals", "M0_H00_095: Liver", "2-Exp Fit of M0_H00_095: Liver", "2-Exp Fit of M0_H00_095: Liver Residuals", "M0_H00_096: Liver", "2-Exp Fit of M0_H00_096: Liver", "2-Exp Fit of M0_H00_096: Liver Residuals", "M0_H00_097: Liver", "2-Exp Fit of M0_H00_097: Liver", "2-Exp Fit of M0_H00_097: Liver Residuals", "M0_H00_098: Liver", "2-Exp Fit of M0_H00_098: Liver", "2-Exp Fit of M0_H00_098: Liver Residuals", "M0_H00_099: Liver", "2-Exp Fit of M0_H00_099: Liver", "2-Exp Fit of M0_H00_099: Liver Residuals", "M0_H00_100: Liver", "2-Exp Fit of M0_H00_100: Liver", "2-Exp Fit of M0_H00_100: Liver Residuals", "M0_H00_101: Liver", "2-Exp Fit of M0_H00_101: Liver", "2-Exp Fit of M0_H00_101: Liver Residuals", "M0_H00_102: Liver", "2-Exp Fit of M0_H00_102: Liver", "2-Exp Fit of M0_H00_102: Liver Residuals", "M0_H00_103: Liver", "2-Exp Fit of M0_H00_103: Liver", "2-Exp Fit of M0_H00_103: Liver Residuals", "M0_H00_104: Liver", "2-Exp Fit of M0_H00_104: Liver", "2-Exp Fit of M0_H00_104: Liver Residuals", "M0_H00_105: Liver", "2-Exp Fit of M0_H00_105: Liver", "2-Exp Fit of M0_H00_105: Liver Residuals", "M0_H00_106: Liver", "2-Exp Fit of M0_H00_106: Liver", "2-Exp Fit of M0_H00_106: Liver Residuals", "M0_H00_107: Liver", "2-Exp Fit of M0_H00_107: Liver", "2-Exp Fit of M0_H00_107: Liver Residuals", "M0_H00_108: Liver", "2-Exp Fit of M0_H00_108: Liver", "2-Exp Fit of M0_H00_108: Liver Residuals", "M0_H00_109: Liver", "2-Exp Fit of M0_H00_109: Liver", "2-Exp Fit of M0_H00_109: Liver Residuals", "M0_H00_110: Liver", "2-Exp Fit of M0_H00_110: Liver", "2-Exp Fit of M0_H00_110: Liver Residuals", "M0_H00_111: Liver", "2-Exp Fit of M0_H00_111: Liver", "2-Exp Fit of M0_H00_111: Liver Residuals", "M0_H00_112: Liver", "2-Exp Fit of M0_H00_112: Liver", "2-Exp Fit of M0_H00_112: Liver Residuals", "M0_H00_113: Liver", "2-Exp Fit of M0_H00_113: Liver", "2-Exp Fit of M0_H00_113: Liver Residuals", "M0_H00_114: Liver", "2-Exp Fit of M0_H00_114: Liver", "2-Exp Fit of M0_H00_114: Liver Residuals", "M0_H00_115: Liver", "2-Exp Fit of M0_H00_115: Liver", "2-Exp Fit of M0_H00_115: Liver Residuals", "M0_H00_116: Liver", "2-Exp Fit of M0_H00_116: Liver", "2-Exp Fit of M0_H00_116: Liver Residuals", "M0_H00_117: Liver", "2-Exp Fit of M0_H00_117: Liver", "2-Exp Fit of M0_H00_117: Liver Residuals", "M0_H00_118: Liver", "2-Exp Fit of M0_H00_118: Liver", "2-Exp Fit of M0_H00_118: Liver Residuals", "M0_H00_119: Liver", "2-Exp Fit of M0_H00_119: Liver", "2-Exp Fit of M0_H00_119: Liver Residuals", "M0_H00_120: Liver", "2-Exp Fit of M0_H00_120: Liver", "2-Exp Fit of M0_H00_120: Liver Residuals", "M0_H00_121: Liver", "2-Exp Fit of M0_H00_121: Liver", "2-Exp Fit of M0_H00_121: Liver Residuals", "M0_H00_122: Liver", "2-Exp Fit of M0_H00_122: Liver", "2-Exp Fit of M0_H00_122: Liver Residuals", "M0_H00_123: Liver", "2-Exp Fit of M0_H00_123: Liver", "2-Exp Fit of M0_H00_123: Liver Residuals", "M0_H00_124: Liver", "2-Exp Fit of M0_H00_124: Liver", "2-Exp Fit of M0_H00_124: Liver Residuals", "M0_H00_125: Liver", "2-Exp Fit of M0_H00_125: Liver", "2-Exp Fit of M0_H00_125: Liver Residuals", "M0_H00_126: Liver", "2-Exp Fit of M0_H00_126: Liver", "2-Exp Fit of M0_H00_126: Liver Residuals", "M0_H00_127: Liver", "2-Exp Fit of M0_H00_127: Liver", "2-Exp Fit of M0_H00_127: Liver Residuals", "M0_H00_128: Liver", "2-Exp Fit of M0_H00_128: Liver", "2-Exp Fit of M0_H00_128: Liver Residuals", "M0_H00_129: Liver", "2-Exp Fit of M0_H00_129: Liver", "2-Exp Fit of M0_H00_129: Liver Residuals", "M0_H00_130: Liver", "2-Exp Fit of M0_H00_130: Liver", "2-Exp Fit of M0_H00_130: Liver Residuals", "M0_H00_131: Liver", "2-Exp Fit of M0_H00_131: Liver", "2-Exp Fit of M0_H00_131: Liver Residuals", "M0_H00_132: Liver", "2-Exp Fit of M0_H00_132: Liver", "2-Exp Fit of M0_H00_132: Liver Residuals", "M0_H00_133: Liver", "2-Exp Fit of M0_H00_133: Liver", "2-Exp Fit of M0_H00_133: Liver Residuals", "M0_H00_134: Liver", "2-Exp Fit of M0_H00_134: Liver", "2-Exp Fit of M0_H00_134: Liver Residuals", "M0_H00_135: Liver", "2-Exp Fit of M0_H00_135: Liver", "2-Exp Fit of M0_H00_135: Liver Residuals", "M0_H00_136: Liver", "2-Exp Fit of M0_H00_136: Liver", "2-Exp Fit of M0_H00_136: Liver Residuals", "M0_H00_137: Liver", "2-Exp Fit of M0_H00_137: Liver", "2-Exp Fit of M0_H00_137: Liver Residuals", "M0_H00_138: Liver", "2-Exp Fit of M0_H00_138: Liver", "2-Exp Fit of M0_H00_138: Liver Residuals", "M0_H00_139: Liver", "2-Exp Fit of M0_H00_139: Liver", "2-Exp Fit of M0_H00_139: Liver Residuals", "M0_H00_140: Liver", "2-Exp Fit of M0_H00_140: Liver", "2-Exp Fit of M0_H00_140: Liver Residuals", "M0_H00_141: Liver", "2-Exp Fit of M0_H00_141: Liver", "2-Exp Fit of M0_H00_141: Liver Residuals", "M0_H00_142: Liver", "2-Exp Fit of M0_H00_142: Liver", "2-Exp Fit of M0_H00_142: Liver Residuals", "M0_H00_143: Liver", "2-Exp Fit of M0_H00_143: Liver", "2-Exp Fit of M0_H00_143: Liver Residuals", "M0_H00_144: Liver", "2-Exp Fit of M0_H00_144: Liver", "2-Exp Fit of M0_H00_144: Liver Residuals", "M0_H00_145: Liver", "2-Exp Fit of M0_H00_145: Liver", "2-Exp Fit of M0_H00_145: Liver Residuals", "M0_H00_146: Liver", "2-Exp Fit of M0_H00_146: Liver", "2-Exp Fit of M0_H00_146: Liver Residuals", "M0_H00_147: Liver", "2-Exp Fit of M0_H00_147: Liver", "2-Exp Fit of M0_H00_147: Liver Residuals", "M0_H00_148: Liver", "2-Exp Fit of M0_H00_148: Liver", "2-Exp Fit of M0_H00_148: Liver Residuals", "M0_H00_149: Liver", "2-Exp Fit of M0_H00_149: Liver", "2-Exp Fit of M0_H00_149: Liver Residuals", "M0_H00_150: Liver", "2-Exp Fit of M0_H00_150: Liver", "2-Exp Fit of M0_H00_150: Liver Residuals", "M0_H00_151: Liver", "2-Exp Fit of M0_H00_151: Liver", "2-Exp Fit of M0_H00_151: Liver Residuals", "M0_H00_152: Liver", "2-Exp Fit of M0_H00_152: Liver", "2-Exp Fit of M0_H00_152: Liver Residuals", "M0_H00_153: Liver", "2-Exp Fit of M0_H00_153: Liver", "2-Exp Fit of M0_H00_153: Liver Residuals", "M0_H00_154: Liver", "2-Exp Fit of M0_H00_154: Liver", "2-Exp Fit of M0_H00_154: Liver Residuals", "M0_H00_155: Liver", "2-Exp Fit of M0_H00_155: Liver", "2-Exp Fit of M0_H00_155: Liver Residuals", "M0_H00_156: Liver", "2-Exp Fit of M0_H00_156: Liver", "2-Exp Fit of M0_H00_156: Liver Residuals", "M0_H00_157: Liver", "2-Exp Fit of M0_H00_157: Liver", "2-Exp Fit of M0_H00_157: Liver Residuals", "M0_H00_158: Liver", "2-Exp Fit of M0_H00_158: Liver", "2-Exp Fit of M0_H00_158: Liver Residuals", "M0_H00_159: Liver", "2-Exp Fit of M0_H00_159: Liver", "2-Exp Fit of M0_H00_159: Liver Residuals", "M0_H00_160: Liver", "2-Exp Fit of M0_H00_160: Liver", "2-Exp Fit of M0_H00_160: Liver Residuals", "M0_H00_161: Liver", "2-Exp Fit of M0_H00_161: Liver", "2-Exp Fit of M0_H00_161: Liver Residuals", "M0_H00_162: Liver", "2-Exp Fit of M0_H00_162: Liver", "2-Exp Fit of M0_H00_162: Liver Residuals", "M0_H00_163: Liver", "2-Exp Fit of M0_H00_163: Liver", "2-Exp Fit of M0_H00_163: Liver Residuals", "M0_H00_164: Liver", "2-Exp Fit of M0_H00_164: Liver", "2-Exp Fit of M0_H00_164: Liver Residuals", "-", "IRF/Reference Decay"]}
  out "Same abscissa array":bool
  in  "Plot Destination":T4
  in  "OK":bool
  in  "Cancel":bool
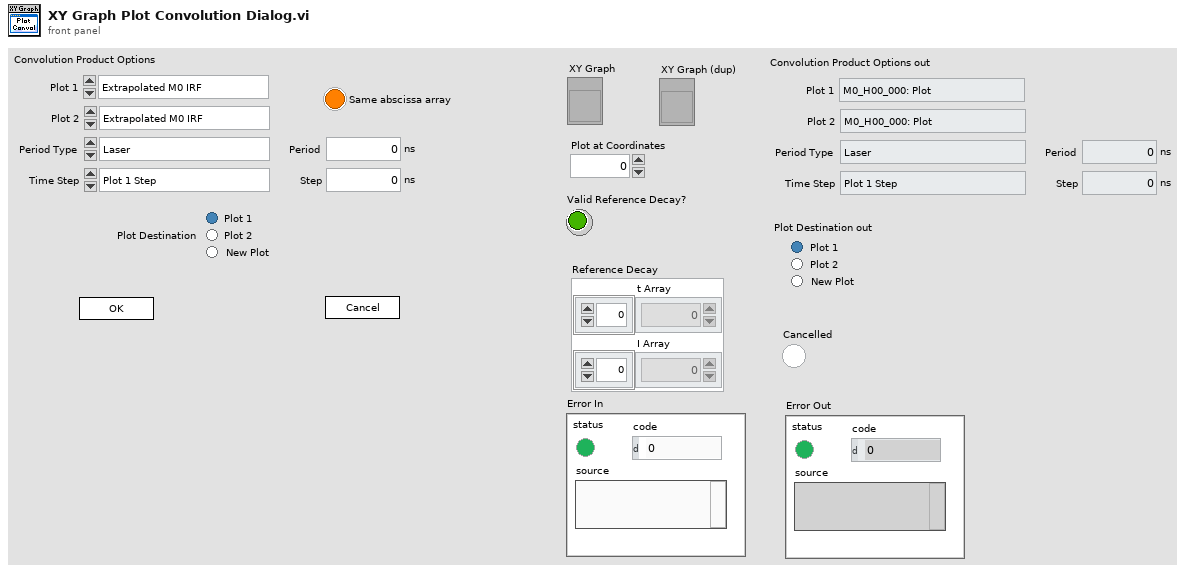
[diagram p1: front panel]
types:
  T1 = typedef "XY Graph Add-Ons.lvlib/XY Graph Convolution Product Options.ctl" = cluster{"Plot 1":u16, "Plot 2":u16, "Period Type":T2, "Period":dbl[unit], "Time Step":T3, "Step":dbl[unit]}
  T2 = typedef "XY Graph Add-Ons.lvlib/XY Graph Convolution Period Type.ctl" = enum16{"Laser", "Plot 1 Duration", "Plot 2 Duration", "User Defined"}
  T3 = typedef "XY Graph Add-Ons.lvlib/XY Graph Convolution Step Type.ctl" = enum16{"Plot 1 Step", "Plot 2 Step", "User Defined"}
  T4 = typedef "Graphs.lvlib/Plot Destination.ctl" = enum32{"Plot 1", "Plot 2", "New Plot"}
  T5 = typedef "XY Graph Add-Ons.lvlib/XY Graph Refnum.ctl" = refnum<vi>
  T6 = typedef "XY Graph Add-Ons.lvlib/XY Plot Data.ctl" = cluster{"X Array":dbl[], "Y Array":dbl[]}
  T7 = typedef "AlliGator Decay Analysis.lvlib/AlliGator Decay Processing.lvlib/AlliGator Convolution Period Type.ctl" = enum16{"Laser", "Plot 1 Duration", "Plot 2 Duration", "User Defined"}
  T8 = typedef "AlliGator Decay Analysis.lvlib/AlliGator Decay Processing.lvlib/AlliGator Convolution Step Type.ctl" = enum16{"Plot 1 Step", "Plot 2 Step", "User Defined"}
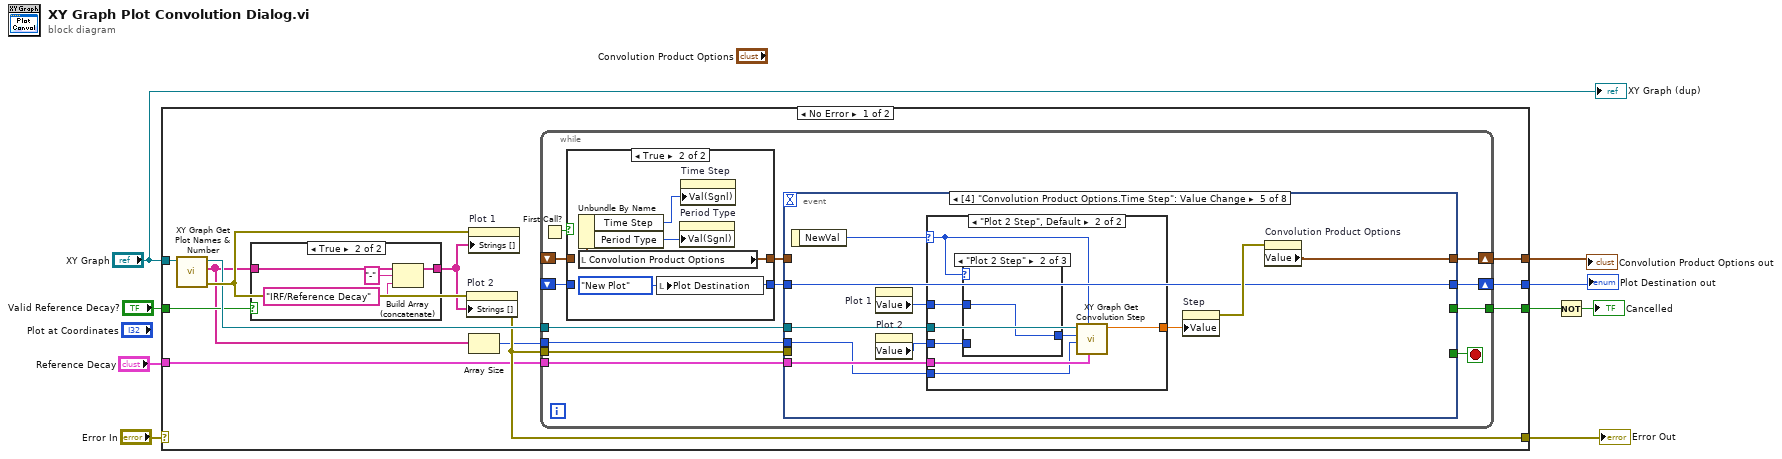
[diagram p0: block diagram]
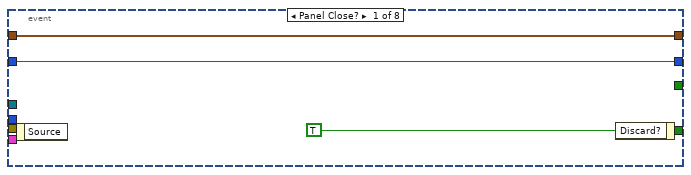
[diagram p3: hidden frame]
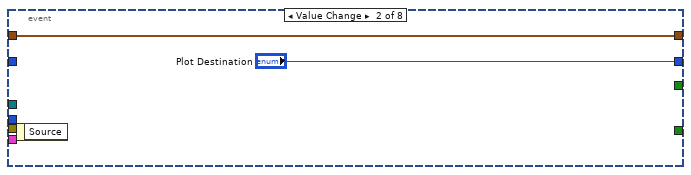
[diagram p4: hidden frame]
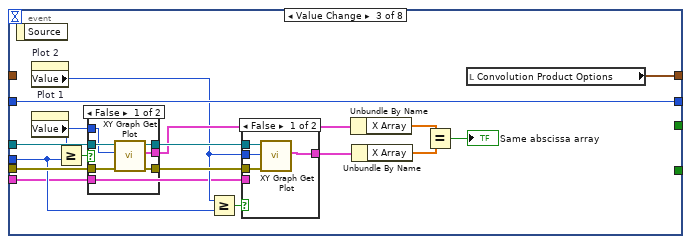
[diagram p5: hidden frame]
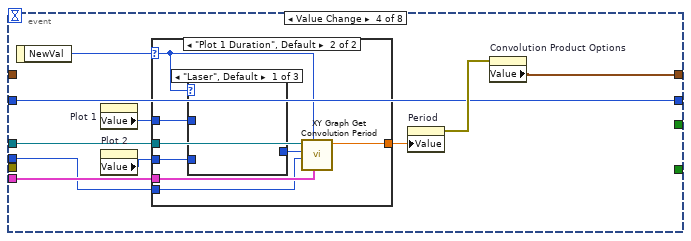
[diagram p8: hidden frame]
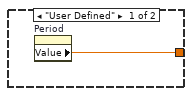
[diagram p9: hidden frame]
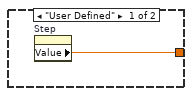
[diagram p12: hidden frame]
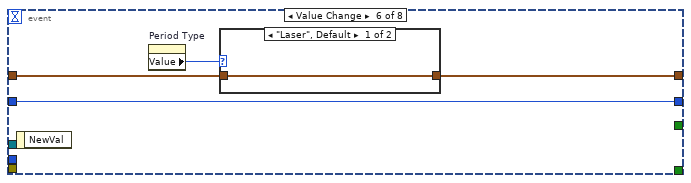
[diagram p15: hidden frame]
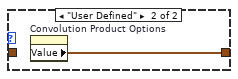
[diagram p16: hidden frame]
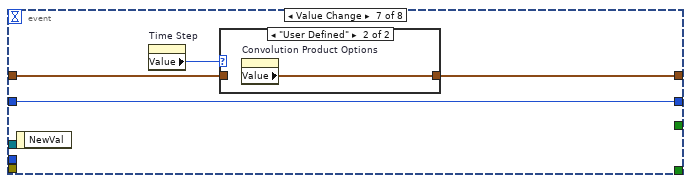
[diagram p17: hidden frame]
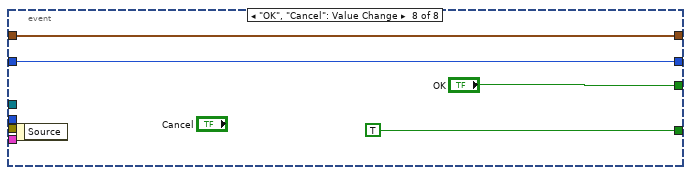
[diagram p19: hidden frame]
diagram:
  n1 = case shown="No Error" "Error In" {
    selector: "Error In" -> [_ w140]
    tunnel: [w21 _] -> w9
    tunnel: [w20 _] -> w3
    tunnel: [w19 _] -> w6
    tunnel: [w16 w140] -> w5
    tunnel: "Valid Reference Decay?" -> [w15 _]
    tunnel: "XY Graph" -> [w14 _]
    tunnel: "Reference Decay" -> [w10 _]
    frame No Error {
      n2 = call "XY Graph Get Plot Names & Number.vi"("XYGraph in"=w14) -> ("error out"=w18:errorcluster, "Plot Names"=w12:string[], "XYGraph out"=w17:T5)  [unwired: 5 in, 3 out]
      n3 = case shown="True" w15 {
        tunnel: w12 -> [w135 w139]
        tunnel: [w135 w138] -> w13
        frame False {
        }
        frame True {
          n4 = Build Array (concatenate)(w139, "-" ("array"), "IRF/Reference Decay" ("array")) -> (w138:string[])
        }
      }
      n5 = property on="Plot 2" class="Ring (strict)"(error in=w18, "Strings []"=w13) -> (error out=w16:errorcluster)  [unwired: 1 in, 1 out]
      n6 = property on="Plot 1" class="Ring (strict)"(error in=w18, "Strings []"=w13) -> ()  [unwired: 1 in, 2 out]
      n7 = Array Size(array=w12) -> (size(s)=w11:i32)
      n8 = while {
        tunnel: [w33] -> w21
        shift-right: [w32] -> w20
        shift-left: _ -> [w27]
        shift-right: [w31] -> w19
        shift-left: _ -> [w26]
        tunnel: w17 -> [w30]
        tunnel: w16 -> [w29]
        tunnel: w11 -> [w23]
        tunnel: w10 -> [w22]
        stop <- w34 stop-if-true
        n9 = First Call?() -> (First Call?: T/F=w28:bool)
        n10 = case shown="True" w28 {
          tunnel: w27 -> [w36 _]
          tunnel: w26 -> [w35 _]
          tunnel: [w36 w39] -> w25
          tunnel: [w35 w40] -> w24
          frame False {
          }
          frame True {
            w40 = Plot_Destination."New Plot" ("Plot Destination")
            n11 = local read "Convolution Product Options"() -> (w39:T1)
            n12 = Unbundle By Name(w39) -> ("Time Step"=w37:T3, "Period Type"=w38:T2)
            n13 = local write "Plot Destination"(w40) -> ()
            n14 = property on="Period Type" class="Enum (strict)"("Val(Sgnl)"=w38) -> ()  [unwired: 2 in, 2 out]
            n15 = property on="Time Step" class="Enum (strict)"("Val(Sgnl)"=w37) -> ()  [unwired: 2 in, 2 out]
          }
        }
        n16 = event shown="[4] \"Convolution Product Options.Time Step\": Value Change" {
          selector: _ -> [_ _ _ _ _ _ _ _]
          dyn-events: _ -> [_ _ _ _ _ _ _ _]
          timeout: _ -> [_ _ _ _ _ _ _ _]
          tunnel: [w43 _ _ _ _ _ _ TRUE ("Discard?")] -> w34
          tunnel: [_ _ _ _ _ _ _ "OK"] -> w33
          tunnel: [w42 w44 w46 w78 w99 w121 w127 w133] -> w32
          tunnel: w25 -> [w42 w44 _ _ _ w120 w126 w133]
          tunnel: [w41 "Plot Destination" w62 w77 w98 w119 w125 w132] -> w31
          tunnel: w24 -> [w41 _ w62 w77 w98 w119 w125 w132]
          tunnel: w30 -> [_ _ w61 w85 w106 _ _ _]
          tunnel: w29 -> [_ _ w60 _ _ _ _ _]
          tunnel: w23 -> [_ _ w49 w81 w102 _ _ _]
          tunnel: w22 -> [_ _ w47 w84 w105 _ _ _]
          event Panel Close? {
            w43 = TRUE ("Discard?")
            n17 = event-data() -> ()  [unwired: 1 in, 1 out]
            n18 = event-data("Discard?"=w43) -> ()  [unwired: 1 in, 1 out]
          }
          event Value Change {
            n19 = event-data() -> ()  [unwired: 1 in, 1 out]
          }
          event Value Change {
            n20 = event-data() -> ()  [unwired: 1 in, 1 out]
            n21 = property on="Plot 2" class="Ring (strict)"() -> ("Value"=w50:u16)  [unwired: 2 in, 2 out]
            n22 = property on="Plot 1" class="Ring (strict)"() -> ("Value"=w52:u16)  [unwired: 2 in, 2 out]
            n23 = Greater Or Equal?(x=w52, y=w49) -> (x >= y?=w51:bool)
            n24 = case shown="False" w51 {
              tunnel: w61 -> [w73 w76]
              tunnel: w60 -> [w72 w74]
              tunnel: [w71 w74] -> w59
              tunnel: [w70 w76] -> w58
              tunnel: [w69 w75] -> w57
              tunnel: w52 -> [w68 _]
              tunnel: w47 -> [_ w75]
              frame False {
                n25 = call "XY Graph Get Plot.vi"("error in (no error)"=w72, "Plot Index (-1: last)"=w68, "XYGraph in"=w73) -> ("error out"=w71:errorcluster, "Plot Data"=w69:T6, "XYGraph out"=w70:T5)  [unwired: 4 in, 2 out]
              }
              frame True {
              }
            }
            n26 = Greater Or Equal?(x=w50, y=w49) -> (x >= y?=w48:bool)
            n27 = case shown="False" w48 {
              tunnel: w59 -> [w66 _]
              tunnel: w58 -> [w65 _]
              tunnel: [w64 w67] -> w56
              tunnel: w50 -> [w63 _]
              tunnel: w47 -> [_ w67]
              frame False {
                n28 = call "XY Graph Get Plot.vi"("error in (no error)"=w66, "Plot Index (-1: last)"=w63, "XYGraph in"=w65) -> ("Plot Data"=w64:T6)  [unwired: 4 in, 4 out]
              }
              frame True {
              }
            }
            n29 = Unbundle By Name(w57) -> ("X Array"=w55:dbl[])
            n30 = Unbundle By Name(w56) -> ("X Array"=w54:dbl[])
            n31 = Equal?(x=w55, y=w54) -> (x = y?=→"Same abscissa array":bool)
            n32 = local read "Convolution Product Options"() -> (w46:T1)
          }
          event Value Change {
            n33 = event-data() -> ("NewVal"=w83:T2)  [unwired: 1 in]
            n34 = property on="Plot 1" class="Ring (strict)"() -> ("Value"=w82:u16)  [unwired: 2 in, 2 out]
            n35 = property on="Plot 2" class="Ring (strict)"() -> ("Value"=w80:u16)  [unwired: 2 in, 2 out]
            n36 = case shown="\"Plot 1 Duration\", Default" w83 {
              selector: w83 -> [_ w89]
              tunnel: [w87 w95] -> w86
              tunnel: w85 -> [_ w94]
              tunnel: w84 -> [_ w93]
              tunnel: w82 -> [_ w91]
              tunnel: w81 -> [_ w90]
              tunnel: w80 -> [_ w88]
              frame "User Defined" {
                n37 = property on="Period" class="DigNum (strict)"() -> ("Value"=w87:dbl[unit])  [unwired: 2 in, 2 out]
              }
              frame "Plot 1 Duration", Default {
                n38 = case shown="\"Laser\", Default" w89 {
                  tunnel: [_ w96 w97] -> w92
                  tunnel: w91 -> [_ w96 _]
                  tunnel: w88 -> [_ _ w97]
                  frame "Laser", Default {
                  }
                  frame "Plot 1 Duration" {
                  }
                  frame "Plot 2 Duration" {
                  }
                }
                n39 = call "XY Graph Get Convolution Period.vi"("Reference Decay"=w93, "Period Type"=w89, "# Plots"=w90, "Selected Plot"=w92, "XYGraph in"=w94) -> ("Period"=w95:dbl[unit])  [unwired: 5 in, 1 out]
              }
            }
            n40 = property on="Period" class="DigNum (strict)"("Value"=w86) -> (error out=w79:errorcluster)  [unwired: 2 in, 1 out]
            n41 = property on="Convolution Product Options" class="Clust (strict)"(error in=w79) -> ("Value"=w78:T1)  [unwired: 1 in, 2 out]
          }
          event Value Change {
            n42 = event-data() -> ("NewVal"=w104:T3)  [unwired: 1 in]
            n43 = property on="Plot 1" class="Ring (strict)"() -> ("Value"=w103:u16)  [unwired: 2 in, 2 out]
            n44 = property on="Plot 2" class="Ring (strict)"() -> ("Value"=w101:u16)  [unwired: 2 in, 2 out]
            n45 = case shown="\"Plot 2 Step\", Default" w104 {
              selector: w104 -> [_ w109]
              tunnel: [w108 w116] -> w107
              tunnel: w106 -> [_ w115]
              tunnel: w105 -> [_ w114]
              tunnel: w103 -> [_ w112]
              tunnel: w102 -> [_ w111]
              tunnel: w101 -> [_ w110]
              frame "User Defined" {
                n46 = property on="Step" class="DigNum (strict)"() -> ("Value"=w108:dbl[unit])  [unwired: 2 in, 2 out]
              }
              frame "Plot 2 Step", Default {
                n47 = case shown="\"Plot 2 Step\"" w109 {
                  tunnel: [_ w117 w118] -> w113
                  tunnel: w112 -> [_ w117 _]
                  tunnel: w110 -> [_ _ w118]
                  frame "Plot 1 Step", Default {
                  }
                  frame "Plot 2 Step" {
                  }
                  frame "User Defined" {
                  }
                }
                n48 = call "XY Graph Get Convolution Step.vi"("Reference Decay"=w114, "Time Step"=w109, "# Plots"=w111, "Selected Plot"=w113, "XYGraph in"=w115) -> ("Step"=w116:dbl[unit])  [unwired: 5 in, 1 out]
              }
            }
            n49 = property on="Step" class="DigNum (strict)"("Value"=w107) -> (error out=w100:errorcluster)  [unwired: 2 in, 1 out]
            n50 = property on="Convolution Product Options" class="Clust (strict)"(error in=w100) -> ("Value"=w99:T1)  [unwired: 1 in, 2 out]
          }
          event Value Change {
            n51 = event-data() -> ()  [unwired: 1 in, 1 out]
            n52 = property on="Period Type" class="Enum (strict)"() -> ("Value"=w122:T7)  [unwired: 2 in, 2 out]
            n53 = case shown="\"Laser\", Default" w122 {
              tunnel: [w123 w124] -> w121
              tunnel: w120 -> [w123 _]
              frame "Laser", Default {
              }
              frame "User Defined" {
                n54 = property on="Convolution Product Options" class="Clust (strict)"() -> ("Value"=w124:T1)  [unwired: 2 in, 2 out]
              }
            }
          }
          event Value Change {
            n55 = event-data() -> ()  [unwired: 1 in, 1 out]
            n56 = property on="Time Step" class="Enum (strict)"() -> ("Value"=w128:T8)  [unwired: 2 in, 2 out]
            n57 = case shown="\"User Defined\"" w128 {
              tunnel: [w129 w130] -> w127
              tunnel: w126 -> [w129 _]
              frame "Plot 1 Step", Default {
              }
              frame "User Defined" {
                n58 = property on="Convolution Product Options" class="Clust (strict)"() -> ("Value"=w130:T1)  [unwired: 2 in, 2 out]
              }
            }
          }
          event "OK", "Cancel": Value Change {
            n59 = event-data() -> ()  [unwired: 1 in, 1 out]
          }
        }
      }
    }
    frame Error {
    }
  }
  "Error Out" <- w5
  "Plot Destination out" <- w6
  "Convolution Product Options out" <- w3
  n60 = Not(x=w9) -> (.not. x?=→"Cancelled":bool)
  "XY Graph (dup)" <- "XY Graph"
